vi "Front Panel.vi"(11 "GUI In":refnum<class "CRD Ringdowns.lvclass">) -> ()   [LabVIEW 2015, in "CRD Ringdowns.lvclass"]
uses:
  CRD Ringdowns.lvclass
  Interface/CRDS/Controls/Ringdown Xctl/Ringdown.xctl
  Interface/CRDS/Controls/Tau Xctl/Tau.xctl
  Reusable/GUI/GUI.lvclass/GUI.ctl
  Reusable/Observer/Observer.lvclass/Observer.ctl
  Reusable/CRDS/Data/Main/CRDS Data.lvclass
  Reusable/CRDS/Data/Cell/CRDS Cell Data.lvclass/CRDS Cell Data.ctl
  Reusable/CRDS/Data/Cell/Read extParam.vi
  Reusable/GUI/Accessors/Read RegEvent.vi
  Reusable/Observer/Read Data Queue.vi
  Reusable/CRDS/Data/Main/Read CellData.vi
  Reusable/Data/Read measTime.vi
  Reusable/CRDS/Data/Cell/Read Ringdowns.vi
  Reusable/Data/Data.lvclass
  Reusable/CRDS/Data/Cell/CRDS Cell Data.lvclass
panel:
  out "tau":cluster{"time":timestamp, "data":sgl[]}(xcontrol)
  out "Ringdown":i16[][][](xcontrol)
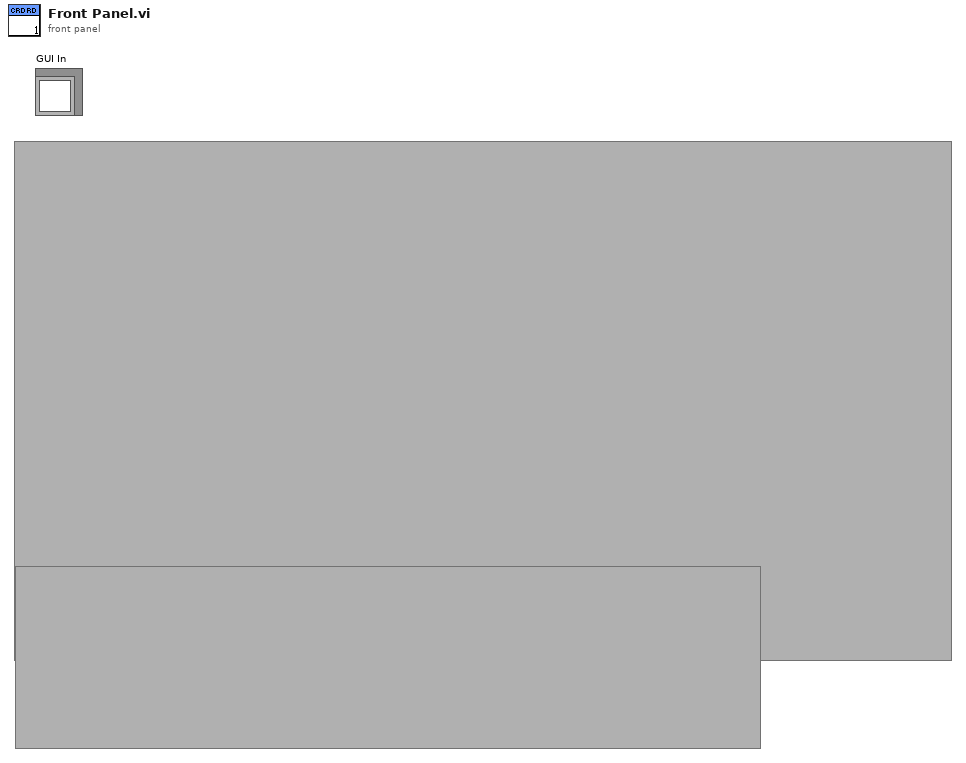
[diagram p1: front panel]
types:
  T1 = cluster{"Name":string, "Line Width":u8, "Line Style":u8, "Color":u32}[]
  T2 = typedef "extparam.ctl" = cluster{"Tau":sgl, "Tau0cor":sgl, "ext":sgl, "extCorr":sgl, "stdevTau":sgl, "eTau":sgl, "taucorr":sgl, "Tau0":sgl, "max":sgl}
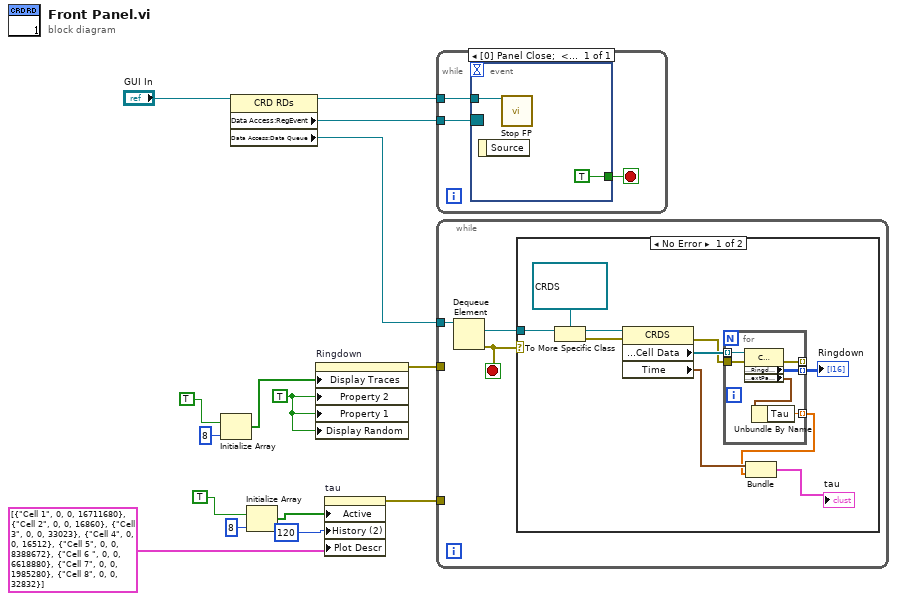
[diagram p0: block diagram]
diagram:
  w8 = TRUE ("Display Data")
  n1 = Initialize Array(TRUE ("Display Data"), 8 ("dimension size")) -> (w7:bool[])
  n2 = property class="CRD RDs"(reference="GUI In") -> (reference out=w12:refnum<class "CRD Ringdowns.lvclass">, "Data Access:RegEvent"=w15:refnum<event-registration>, "Data Access:Data Queue"=w14:refnum<queue>)  [unwired: 1 in, 1 out]
  n3 = Initialize Array(TRUE, 8 ("dimension size")) -> (w4:bool[])
  n4 = property on="Ringdown" class="Ringdown (strict)"("Display Traces"=w7, "Property 2"=w8, "Property 1"=w8, "Display Random"=w8) -> (error out=w11:errorcluster)  [unwired: 2 in, 1 out]
  n5 = property on="tau" class="1D Buffer (strict)"("Active"=w4, "History (2)"=u16 120 ("History"), "Plot Descr"=T1 [{"Name"="Cell 1", "Line Width"=0, "Line Style"=0, "Color"=16711680}, {"Name"="Cell 2", "Line Width"=0, "Line Style"=0, "Color"=16860}, {"Name"="Cell 3", "Line Width"=0, "Line Style"=0, "Color"=33023}, {"Name"="Cell 4", "Line Width"=0, "Line Style"=0, "Color"=16512}, {"Name"="Cell 5", "Line Width"=0, "Line Style"=0, "Color"=8388672}, {"Name"="Cell 6 ", "Line Width"=0, "Line Style"=0, "Color"=6618880}, {"Name"="Cell 7", "Line Width"=0, "Line Style"=0, "Color"=1985280}, {"Name"="Cell 8", "Line Width"=0, "Line Style"=0, "Color"=32832}]) -> (error out=w3:errorcluster)  [unwired: 2 in, 1 out]
  n6 = while {
    tunnel: w15 -> [w17]
    tunnel: w12 -> [w16]
    stop <- w18 stop-if-true
    n7 = event shown="[0] Panel Close;  <True>: User Event" {
      selector: w17 -> [_]
      dyn-events: _ -> [_]
      timeout: _ -> [_]
      tunnel: [TRUE] -> w18
      tunnel: w16 -> [w19]
      event Panel Close; User Event {
        n8 = event-data() -> ()  [unwired: 1 in, 1 out]
        n9 = call-dynamic "Stop FP.vi"("GUI in"=w19) -> ()  [unwired: 9 in, 2 out]
      }
    }
  }
  n10 = while {
    tunnel: w14 -> [w23]
    tunnel: w11 -> [_]
    tunnel: w3 -> [_]
    stop <- w22 stop-if-true
    n11 = Dequeue Element(queue=w23) -> (element=w21:refnum<data-value>, error out=w22:errorcluster)  [unwired: 2 in, 2 out]
    n12 = case shown="No Error" w22 {
      tunnel: w21 -> [w31 _]
      frame No Error {
        n13 = To More Specific Class(target class=refnum<data-value> refnum ("data value reference"), reference=w31) -> (specific class reference=w30:refnum<data-value>, error out=w27:errorcluster)  [unwired: 1 in]
        n14 = property class="CRDS"(reference=w30, error in=w27) -> (error out=w32:errorcluster, "Data Access:Cell Data"=w33:refnum<class "CRDS Cell Data.lvclass">[], "Time"=w26:timestamp)  [unwired: 1 out]
        n15 = for {
          tunnel: w33 -> [w39] mode=indexing
          tunnel: [w38] -> w28 mode=indexing
          tunnel: [w37] -> _ mode=indexing
          tunnel: w32 -> [w36]
          tunnel: [w34] -> w25 mode=indexing
          n16 = property class="CRDS Cell"(reference=w39, error in=w36) -> (error out=w37:errorcluster, "Data Access:Ringdowns"=w38:i16[][], "Data Access:extParam"=w35:T2)  [unwired: 1 out]
          n17 = Unbundle By Name(w35) -> ("Tau"=w34:sgl)
        }
        "Ringdown" <- w28
        n18 = Bundle("Time"=w26, w25) -> (→"tau":cluster{"Time":timestamp, sgl[]})  [unwired: 1 in]
      }
      frame Error {
      }
    }
  }
